vi "4155C Config VSU2 Stress.vi"(2 "error in (no error)":errorcluster, 3 "VSU2":dbl min=0.0 max=100000000000.0 format="%.15e", 4 "Display on/off":bool, 5 "VISA session":refnum<visa-resource-name>) -> (0 "error out":errorcluster, 1 "dup VISA resource name":refnum<visa-resource-name>)   [LabVIEW 2016]
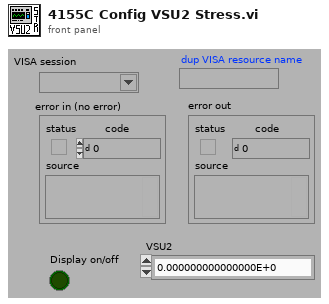
[diagram p1: front panel]
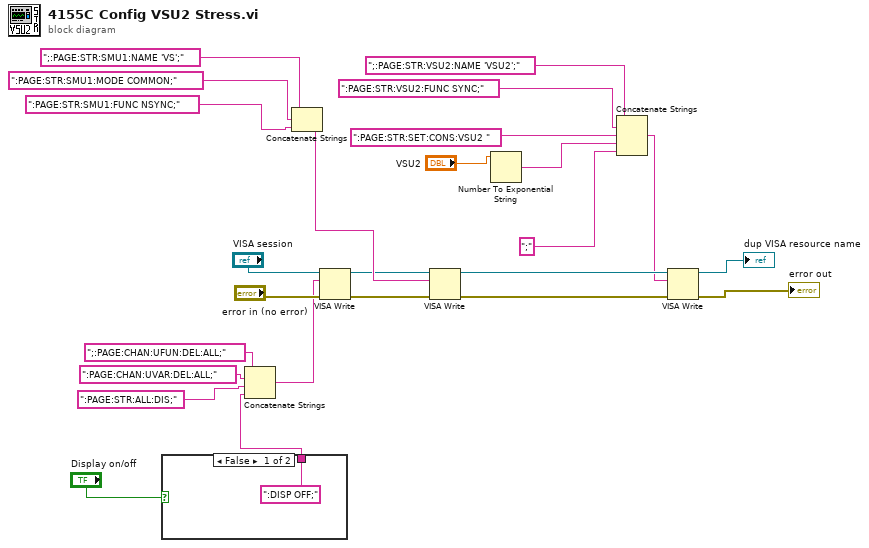
[diagram p0: block diagram]
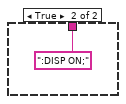
[diagram p2: hidden frame]
diagram:
  n1 = case shown="False" "Display on/off" {
    tunnel: [":DISP OFF;" ("write buffer (\"\")") ":DISP ON;" ("write buffer (\"\")")] -> w19
    frame False {
    }
    frame True {
    }
  }
  n2 = Concatenate Strings(";:PAGE:CHAN:UFUN:DEL:ALL;", ":PAGE:CHAN:UVAR:DEL:ALL;", ":PAGE:STR:ALL:DIS;", w19) -> (w20:string)
  n3 = Concatenate Strings(";:PAGE:STR:SMU1:NAME 'VS';", ":PAGE:STR:SMU1:MODE COMMON;", ":PAGE:STR:SMU1:FUNC NSYNC;") -> (w9:string)
  n4 = VISA Write(VISA resource name="VISA session", write buffer=w20, error in (no error)="error in (no error)") -> (VISA resource name out=w8:refnum<visa-resource-name>, error out=w7:errorcluster)  [unwired: 1 out]
  n5 = VISA Write(VISA resource name=w8, write buffer=w9, error in (no error)=w7) -> (VISA resource name out=w25:refnum<visa-resource-name>, error out=w24:errorcluster)  [unwired: 1 out]
  n6 = Number To Exponential String(number="VSU2") -> (E-format string=w11:string)  [unwired: 3 in]
  n7 = Concatenate Strings(";:PAGE:STR:VSU2:NAME 'VSU2';", ":PAGE:STR:VSU2:FUNC SYNC;", ":PAGE:STR:SET:CONS:VSU2 ", w11, ";" ("Substring")) -> (w6:string)
  n8 = VISA Write(VISA resource name=w25, write buffer=w6, error in (no error)=w24) -> (VISA resource name out=→"dup VISA resource name":refnum<visa-resource-name>, error out=→"error out":errorcluster)  [unwired: 1 out]
